vi "MyServer.vi"(8 "error in (no error)":errorcluster, 11 "Stop event":refnum<user-event>) -> (0 "error server":errorcluster)   [LabVIEW 2018]
uses:
  Server/Server class/Server.lvclass/Server.ctl
  Server/Server class/Server.lvclass
  C:/Users/jdeboeck/Source/Repos/LV-MQTT-Broker/source/MQTT_Base/MQTT_Base.lvclass
  MQTT_Base/MQTT_Base.lvclass
panel:
  in  "stop":bool
  out "NbConnections":u32
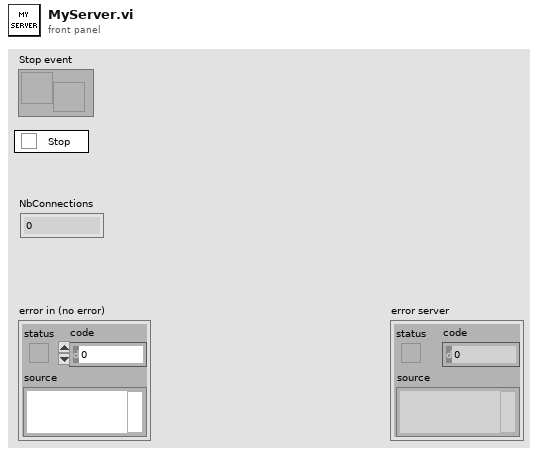
[diagram p1: front panel]
types:
  T1 = typedef "MQTT Server.lvlib/Server.lvclass/Public Events -- cluster.ctl" = cluster{"NbConnections":refnum<user-event>}
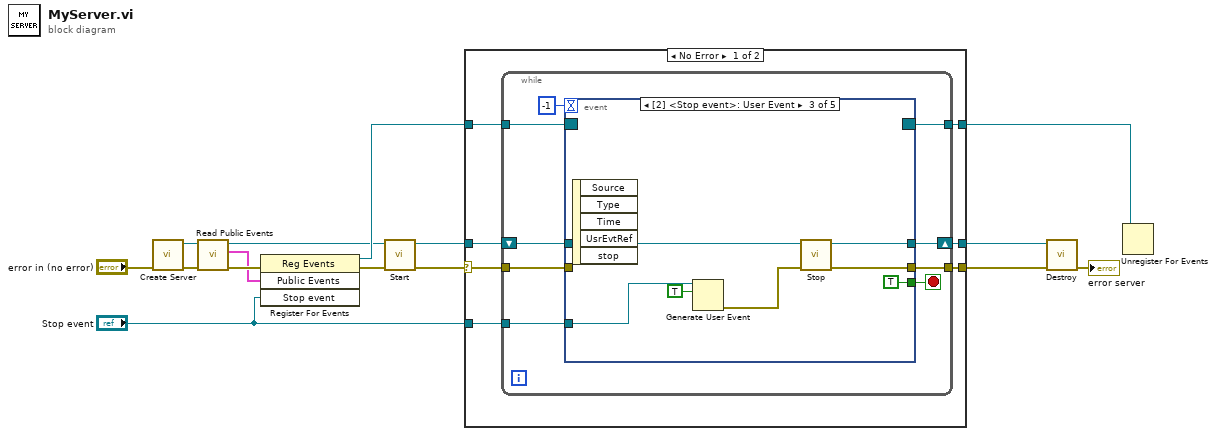
[diagram p0: block diagram]
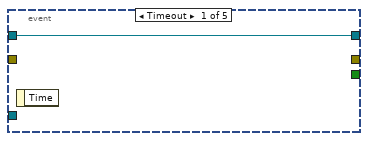
[diagram p2: hidden frame]
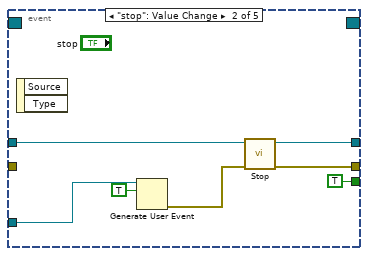
[diagram p3: hidden frame]
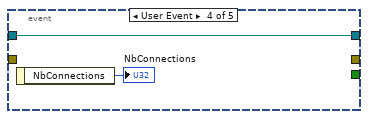
[diagram p4: hidden frame]
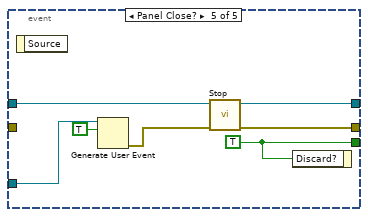
[diagram p5: hidden frame]
diagram:
  n1 = call "Create Server.vi"("error in (no error)"="error in (no error)") -> ("error out"=w13:errorcluster, "Server"=w14:refnum<class "Server.lvclass">)  [unwired: 9 in]
  n2 = call "Read Public Events.vi"("error in (no error)"=w13, "Server in"=w14) -> ("error out"=w12:errorcluster, "Public Events"=w11:T1, "Server out"=w8:refnum<class "Server.lvclass">)  [unwired: 7 in]
  n3 = register-events(error in=w12, w11, "Stop event") -> (reference out=w10:refnum<event-registration>, error out=w6:errorcluster)  [unwired: 1 in]
  n4 = call "Start.vi"("error in (no error)"=w6, "MQTT_Base in"=w8) -> ("error out"=w4:errorcluster, "MQTT_Base out"=w7:refnum<class "Server.lvclass">)  [unwired: 7 in, 1 out]
  n5 = case shown="No Error" w4 {
    selector: w4 -> [w17 w56]
    tunnel: w7 -> [w22 w58]
    tunnel: [w21 w58] -> w15
    tunnel: w10 -> [w20 w57]
    tunnel: [w19 w57] -> w9
    tunnel: [w18 w56] -> w5
    tunnel: "Stop event" -> [w16 _]
    frame No Error {
      n6 = while {
        shift-right: [w28] -> w21
        shift-left: w22 -> [w30]
        tunnel: w20 -> [w27]
        tunnel: [w26] -> w19
        tunnel: [w25] -> w18
        tunnel: w17 -> [w24]
        tunnel: w16 -> [w23]
        stop <- w29 stop-if-true
        n7 = event shown="[2] <Stop event>: User Event" {
          selector: w27 -> [_ _ _ _ _]
          dyn-events: [_ _ _ _ _] -> w26
          timeout: -1 -> [_ _ _ _ _]
          tunnel: w30 -> [w32 w39 w46 w48 w55]
          tunnel: [_ TRUE ("Discard?") TRUE ("Discard?") _ w54] -> w29
          tunnel: [w32 w38 w45 w48 w53] -> w28
          tunnel: [_ w37 w44 _ w52] -> w25
          tunnel: w24 -> [_ _ _ _ _]
          tunnel: w23 -> [_ w34 w41 _ w49]
          event Timeout {
            n8 = event-data() -> ()  [unwired: 1 in, 1 out]
          }
          event "stop": Value Change {
            n9 = event-data() -> ()  [unwired: 1 in, 2 out]
            n10 = Generate User Event(user event=w34, event data cluster=TRUE ("event data")) -> (error out=w33:errorcluster)  [unwired: 2 in, 1 out]
            n11 = call "Stop.vi"("error in (no error)"=w33, "MQTT_Base in"=w39) -> ("error out"=w37:errorcluster, "MQTT_Base out"=w38:refnum<class "Server.lvclass">)  [unwired: 7 in, 1 out]
          }
          event User Event {
            n12 = event-data() -> ()  [unwired: 1 in, 5 out]
            n13 = Generate User Event(user event=w41, event data cluster=TRUE ("event data")) -> (error out=w40:errorcluster)  [unwired: 2 in, 1 out]
            n14 = call "Stop.vi"("error in (no error)"=w40, "MQTT_Base in"=w46) -> ("error out"=w44:errorcluster, "MQTT_Base out"=w45:refnum<class "Server.lvclass">)  [unwired: 7 in, 1 out]
          }
          event User Event {
            n15 = event-data() -> ("NbConnections"=→"NbConnections":u32)  [unwired: 1 in]
          }
          event Panel Close? {
            w54 = TRUE ("Discard?")
            n16 = event-data() -> ()  [unwired: 1 in, 1 out]
            n17 = Generate User Event(user event=w49, event data cluster=TRUE ("event data")) -> (error out=w50:errorcluster)  [unwired: 2 in, 1 out]
            n18 = call "Stop.vi"("error in (no error)"=w50, "MQTT_Base in"=w55) -> ("error out"=w52:errorcluster, "MQTT_Base out"=w53:refnum<class "Server.lvclass">)  [unwired: 7 in, 1 out]
            n19 = event-data("Discard?"=w54) -> ()  [unwired: 1 in, 1 out]
          }
        }
      }
    }
    frame Error {
    }
  }
  n20 = call "Destroy.vi"("error in (no error)"=w5, "MQTT_Base in"=w15) -> ("error out"=→"error server":errorcluster)  [unwired: 8 in, 1 out]
  n21 = Unregister For Events(event registration refnum=w9) -> ()  [unwired: 1 in, 1 out]
